vi "zad2.vi"() -> ()   [LabVIEW 2017]
uses:
  <vilib>/express/express arith-compare/Formula/XNode/ExpressFormulaBlockNode.xnode
panel:
  out "XY Graph":cluster{dbl[], dbl[]}[](graph)
  out "error out":errorcluster
  in  "error in (no error)":errorcluster
  in  "Zakres":cluster{"Min":dbl, "Max":dbl, "Krok":dbl}
  in  "Wspo³czynniki wielomianu":cluster{"a":dbl, "b":dbl, "c":dbl, "d":dbl}
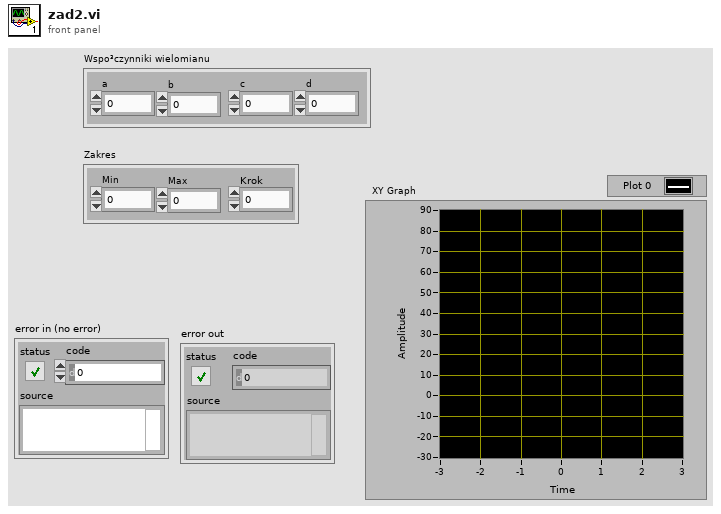
[diagram p1: front panel]
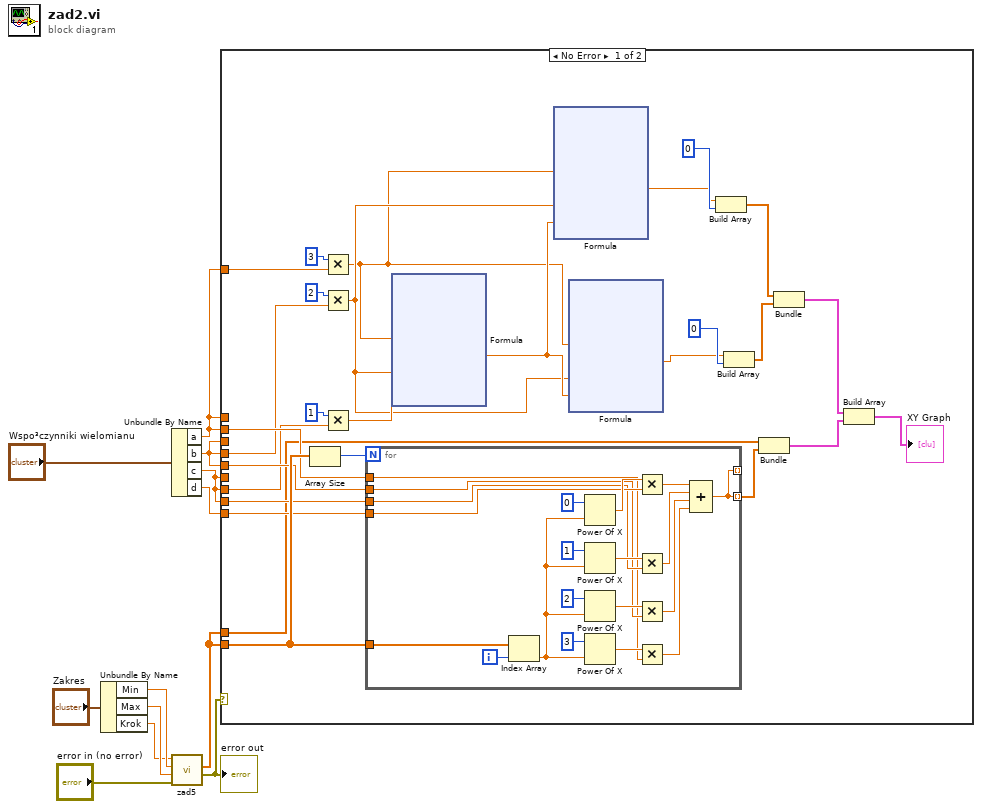
[diagram p0: block diagram]
diagram:
  n1 = Unbundle By Name("Zakres") -> ("Min"=w10:dbl, "Max"=w9:dbl, "Krok"=w8:dbl)
  n2 = Unbundle By Name("Wspo³czynniki wielomianu") -> ("a"=w3:dbl, "b"=w2:dbl, "c"=w1:dbl, "d"=w5:dbl)
  n3 = call "zad5.vi"("error in (no error)"="error in (no error)", "Max"=w9, "Min"=w10, "Delta"=w8) -> ("error out"=w6:errorcluster, "Array"=w4:dbl[])  [unwired: 6 in]
  "error out" <- w6
  n4 = case shown="No Error" w6 {
    tunnel: w4 -> [w39 _]
    tunnel: w5 -> [w38 _]
    tunnel: w1 -> [w37 _]
    tunnel: w2 -> [w36 _]
    tunnel: w3 -> [w35 _]
    tunnel: w4 -> [w26 _]
    tunnel: w3 -> [_ _]
    tunnel: w2 -> [_ _]
    tunnel: w1 -> [_ _]
    tunnel: w3 -> [w30 _]
    tunnel: w2 -> [w29 _]
    tunnel: w1 -> [w28 _]
    frame No Error {
      n5 = Array Size(array=w39) -> (size(s)=w34:i32)
      n6 = Multiply(x=3, y=w30) -> (x*y=w22:dbl)
      n7 = Multiply(x=2, y=w29) -> (x*y=w23:dbl)
      n8 = Multiply(x=1, y=w28) -> (x*y=w27:dbl)
      n9 = for {
        N: w34 -> [_]
        tunnel: w39 -> [w95]
        tunnel: w38 -> [w92]
        tunnel: w37 -> [w88]
        tunnel: w36 -> [w87]
        tunnel: w35 -> [w86]
        tunnel: [w76] -> _ mode=indexing
        tunnel: [w76] -> w25 mode=indexing
        i -> [w81]
        n10 = Index Array(array=w95, index=w81) -> (element=w94:dbl)
        n11 = Power Of X(1:w94, 2:0) -> (0:w93:dbl)
        n12 = Power Of X(1:w94, 2:1) -> (0:w91:dbl)
        n13 = Power Of X(1:w94, 2:2) -> (0:w90:dbl)
        n14 = Power Of X(1:w94, 2:3) -> (0:w89:dbl)
        n15 = Multiply(x=w93, y=w92) -> (x*y=w85:dbl)
        n16 = Multiply(x=w91, y=w88) -> (x*y=w84:dbl)
        n17 = Multiply(x=w90, y=w87) -> (x*y=w83:dbl)
        n18 = Multiply(x=w89, y=w86) -> (x*y=w82:dbl)
        n19 = Compound Arithmetic op=ADD(w85, w84, w83, w82) -> (w76:dbl)
      }
      n20 = xnode "Formula"("a"=w22, "b"=w23, "c"=w27) -> ("Result"=w24:dbl)  [unwired: 1 in, 1 out]
      n21 = xnode "Formula"("a"=w22, "b"=w23, "delta"=w24) -> ("Result"=w15:dbl)  [unwired: 1 in, 1 out]
      n22 = xnode "Formula"("a"=w22, "b"=w23, "delta"=w24) -> ("Result"=w13:dbl)  [unwired: 1 in, 1 out]
      n23 = Build Array(w15, 0) -> (w21:dbl[])
      n24 = Build Array(w13, 0) -> (w20:dbl[])
      n25 = Bundle("Array"=w26, w25) -> (w18:cluster{"Array":dbl[], dbl[]})  [unwired: 1 in]
      n26 = Bundle(w21, w20) -> (w17:cluster{dbl[], dbl[]})  [unwired: 1 in]
      n27 = Build Array(w17, w18) -> (→"XY Graph":cluster{"Array":dbl[], dbl[]}[])
    }
    frame Error {
    }
  }
